vi "PathPlanner_PathConstraints_Equals.vi"(9 "Other PathPlannerConstraints":T1, 11 "PathPlannerConstraints":T1) -> (3 "Equal":bool)   [LabVIEW 2019, in "PathPlanner24.lvlib"]
doc: "/**\n * Create a new path constraints object\n *\n * @param maxVelocityMps Max linear velocity (M/S)\n * @param maxAccelerationMpsSq Max linear acceleration (M/S^2)\n * @param maxAngularVelocityRps Max angular velocity (Rad/S)\n * @param maxAngularAccelerationRpsSq Max angular acceleration (Rad/S^2)\n */"
uses:
  PathPlanner24.lvlib
  TypeDef/PathPlannerPathConstraints.ctl
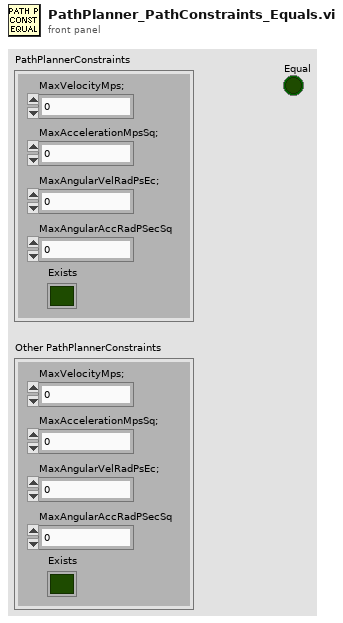
[diagram p1: front panel]
types:
  T1 = typedef "PathPlanner24.lvlib/PathPlannerPathConstraints.ctl" = cluster{"MaxVelocityMps;":dbl, "MaxAccelerationMpsSq;":dbl, "MaxAngularVelRadPsEc;":dbl, "MaxAngularAccRadPSecSq":dbl, "Exists":bool}
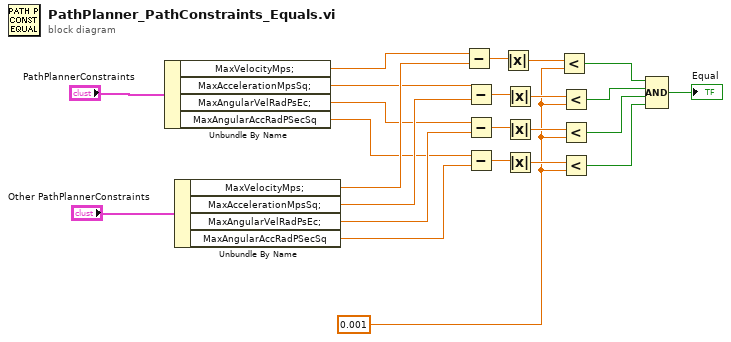
[diagram p0: block diagram]
diagram:
  w1 = 0.001 ("y")
  n1 = Unbundle By Name("PathPlannerConstraints") -> ("MaxVelocityMps;"=w22:dbl, "MaxAccelerationMpsSq;"=w12:dbl, "MaxAngularVelRadPsEc;"=w10:dbl, "MaxAngularAccRadPSecSq"=w8:dbl)
  n2 = Unbundle By Name("Other PathPlannerConstraints") -> ("MaxVelocityMps;"=w21:dbl, "MaxAccelerationMpsSq;"=w11:dbl, "MaxAngularVelRadPsEc;"=w9:dbl, "MaxAngularAccRadPSecSq"=w7:dbl)
  n3 = Subtract(x=w22, y=w21) -> (x-y=w20:dbl)
  n4 = Subtract(x=w12, y=w11) -> (x-y=w18:dbl)
  n5 = Subtract(x=w10, y=w9) -> (x-y=w16:dbl)
  n6 = Subtract(x=w8, y=w7) -> (x-y=w14:dbl)
  n7 = Absolute Value(x=w20) -> (abs(x)=w19:dbl)
  n8 = Absolute Value(x=w18) -> (abs(x)=w17:dbl)
  n9 = Absolute Value(x=w16) -> (abs(x)=w15:dbl)
  n10 = Absolute Value(x=w14) -> (abs(x)=w13:dbl)
  n11 = Less?(x=w19, y=w1) -> (x < y?=w6:bool)
  n12 = Less?(x=w17, y=w1) -> (x < y?=w5:bool)
  n13 = Less?(x=w15, y=w1) -> (x < y?=w4:bool)
  n14 = Less?(x=w13, y=w1) -> (x < y?=w3:bool)
  n15 = Compound Arithmetic op=AND(w6, w5, w4, w3) -> (→"Equal":bool)
